vi "Average Sectors.vi"   [LabVIEW 2013]
uses:
  Globals/Accumulated Sector Intensity.vi
  <vilib>/rvi/Memory/Memory_Emulation/nirvimemoryFastEmulationFpgaImpl.vi
  <instcachedir>/0/nirvimemoryFastEmulationFpgaImpl_5FBAB50466BC4C939F684F8805638BFC.lvgen/nirvimemoryFastEmulationFpgaImpl_5FBAB50466BC4C939F684F8805638BFC_012.vi
  <vilib>/rvi/DataTransferAndStorage/Container/Common/niFpgaContainerGetUniqueNameForEmu.vi
  <vilib>/rvi/Memory/Memory_Emulation/nirvimemoryFastEmulation.vi
  <vilib>/rvi/Memory/Memory_Emulation/nirvimemoryEmulation.vi
  Globals/Sector Parameter Global.vi
  <vilib>/rvi/FIFO/Fifo_Resource/nirvififoEmulationWriteFpgaImpl.vi
  <vilib>/rvi/DataTransferAndStorage/Container/XNode/niFpgaContainer.xnode
  <vilib>/rvi/FIFO/Fifo_Resource/nirvififoEmulationWrite.vi
types:
  T1 = cluster{"Accumulated Intensity":fxp<+,20,20>, "Count":fxp<+,12,12>}[]
  T2 = cluster{"Accumulated Intensity":fxp<+,20,20>, "Count":fxp<+,12,12>}
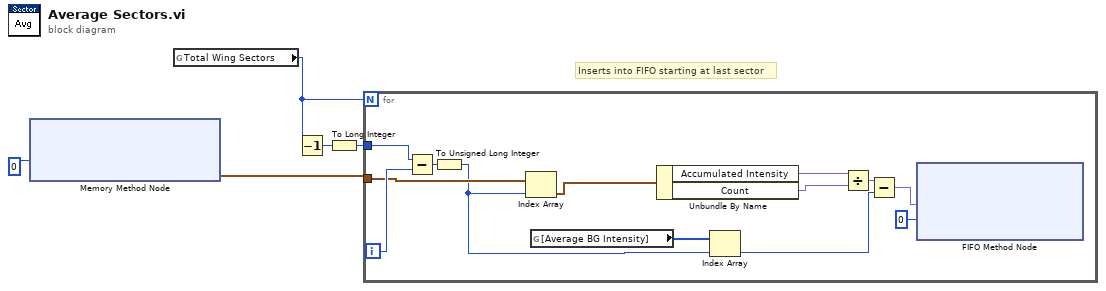
[diagram p0: block diagram]
diagram:
  # "Inserts into FIFO starting at last sector"
  n1 = xnode ("Memory Method Node")("Address"=u32 0) -> ("Data"=w1:T1)  [unwired: 1 in, 1 out]
  n2 = global read "Accumulated Sector Intensity.vi" "Total Wing Sectors"() -> (w3:u8)
  n3 = Decrement(x=w3) -> (x-1=w5:u8)
  n4 = To Long Integer(number=w5) -> (32bit integer=w4:i32)
  n5 = for {
    N: w3 -> [_]
    tunnel: w4 -> [w13]
    tunnel: w1 -> [w10]
    i -> [w11]
    n6 = Subtract(x=w13, y=w11) -> (x-y=w12:i32)
    n7 = To Unsigned Long Integer(number=w12) -> (unsigned 32bit integer=w9:u32)
    n8 = Index Array(array=w10, index=w9) -> (element=w8:T2)
    n9 = global read "Sector Parameter Global.vi" "[Average BG Intensity]"() -> (w17:u8[])
    n10 = Unbundle By Name(w8) -> ("Accumulated Intensity"=w7:fxp<+,20,20>, "Count"=w6:fxp<+,12,12>)
    n11 = Index Array(array=w17, index=w9) -> (element=w15:u8)
    n12 = Divide(x=w7, y=w6) -> (x/y=w16:fxp<+,8,8>)
    n13 = Subtract(x=w16, y=w15) -> (x-y=w14:fxp<+/-,9,9>)
    n14 = xnode ("FIFO Method Node")("Element"=w14, "Timeout"=0) -> ()  [unwired: 1 in, 2 out]
  }
